vi "box_array.vi"(5 "Box Width":dbl=2.5 format="%.2f", 7 "X position":dbl=5.0 format="%.2f", 9 "Lower Quartile (LQ)":dbl=1.5 format="%.2f", 10 "Median":dbl=3.0 format="%.2f", 11 "Upper Quartile (UQ)":dbl=4.5 format="%.2f") -> (3 "XY Graph":cluster{dbl[], dbl[]}(graph))   [LabVIEW 2021, in "statistics.lvlib"]
uses:
  statistics.lvlib
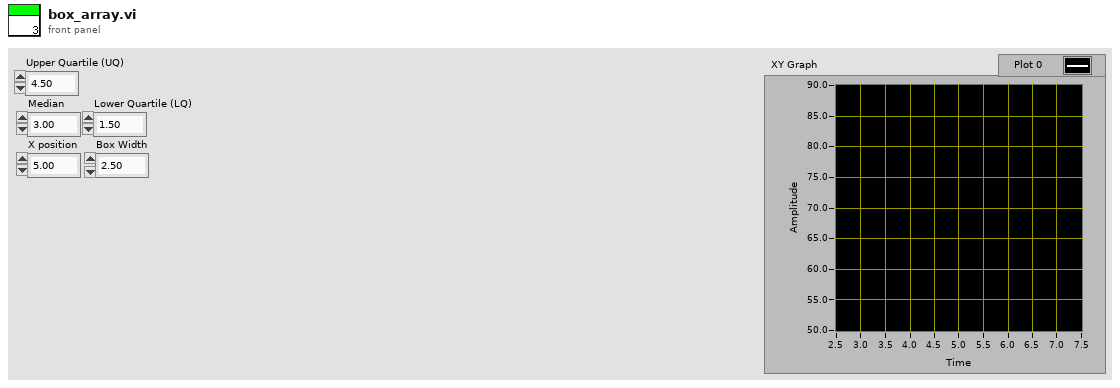
[diagram p1: front panel]
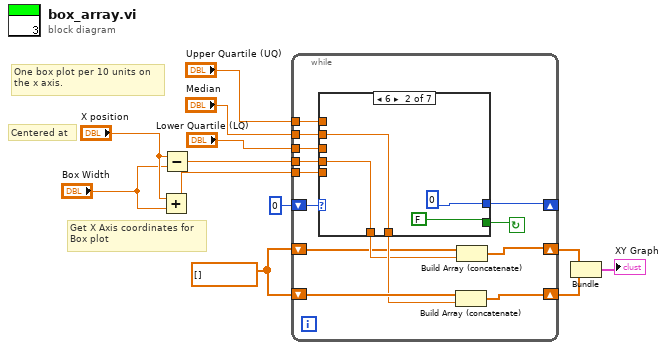
[diagram p0: block diagram]
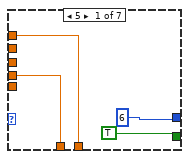
[diagram p2: hidden frame]
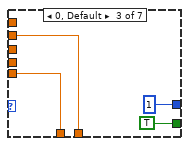
[diagram p3: hidden frame]
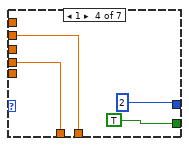
[diagram p4: hidden frame]
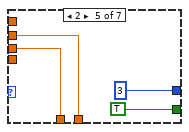
[diagram p5: hidden frame]
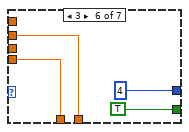
[diagram p6: hidden frame]
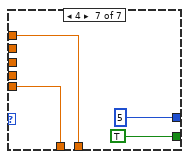
[diagram p7: hidden frame]
diagram:
  w3 = dbl[] []
  # "Centered at"
  # "One box plot per 10 units on\nthe x axis."
  # "Get X Axis coordinates for\nBox plot"
  n1 = Add(x="X position", y="Box Width") -> (x+y=w4:dbl)
  n2 = Subtract(x="X position", y="Box Width") -> (x-y=w5:dbl)
  n3 = while {
    shift-right: [w13] -> w8
    shift-left: w3 -> [w14]
    shift-right: [w17] -> w7
    shift-left: w3 -> [w18]
    shift-right: [w26] -> _
    shift-left: 0 -> [w25]
    tunnel: "Upper Quartile (UQ)" -> [w23]
    tunnel: "Median" -> [w22]
    tunnel: "Lower Quartile (LQ)" -> [w21]
    tunnel: w5 -> [w20]
    tunnel: w4 -> [w19]
    stop <- w24 continue-if-true
    n4 = case shown="6" w25 {
      tunnel: [6 0 1 2 3 4 5] -> w26
      tunnel: [TRUE FALSE TRUE TRUE TRUE TRUE TRUE] -> w24
      tunnel: w23 -> [w28 _ _ _ _ _ w51]
      tunnel: w22 -> [_ w32 w35 w39 _ _ _]
      tunnel: w21 -> [_ _ _ _ w43 w47 _]
      tunnel: w20 -> [w29 w33 _ w40 w44 _ _]
      tunnel: w19 -> [_ _ w36 _ _ w48 w52]
      tunnel: [w29 w33 w36 w40 w44 w48 w52] -> w15
      tunnel: [w28 w32 w35 w39 w43 w47 w51] -> w16
      frame 5 {
      }
      frame 6 {
      }
      frame 0, Default {
      }
      frame 1 {
      }
      frame 2 {
      }
      frame 3 {
      }
      frame 4 {
      }
    }
    n5 = Build Array (concatenate)(w18, w16) -> (w17:dbl[])
    n6 = Build Array (concatenate)(w14, w15) -> (w13:dbl[])
  }
  n7 = Bundle(w8, w7) -> (→"XY Graph":cluster{dbl[], dbl[]})  [unwired: 1 out]
